vi "ConvertNumericChannelsToStringChannels.vi"(0 "Channels (In)":i32[](array[numeric])) -> (4 "Channels (A:B:C:D...) (Out)":string)   [LabVIEW 2015]
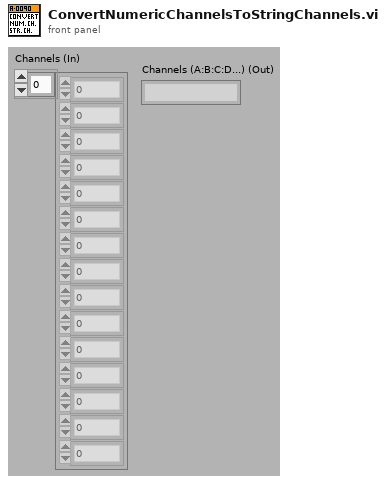
[diagram p1: front panel]
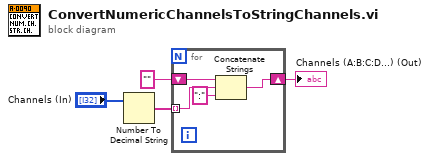
[diagram p0: block diagram]
diagram:
  n1 = Number To Decimal String(number="Channels (In)") -> (decimal integer string=w3:string[])  [unwired: 1 in]
  n2 = for {
    tunnel: w3 -> [w5] mode=indexing
    shift-right: [w7] -> w2
    shift-left: "" -> [w8]
    n3 = Concatenate Strings(w8, w5, ":" ("string")) -> (w7:string)
  }
  "Channels (A:B:C:D...) (Out)" <- w2
